vi "_FPGA_ConjSelector.vi"(0 "Conj.InitCyc*2^32":u32, 1 "ConjArr":cluster{"Ratio*2^15":u16, "CycleDiff":u64}[](array[cluster])=[{"Ratio*2^15"=0, "CycleDiff"=0}, {"Ratio*2^15"=0, "CycleDiff"=0}, {"Ratio*2^15"=0, "CycleDiff"=0}, {"Ratio*2^15"=0, "CycleDiff"=0}, {"Ratio*2^15"=0, "CycleDiff"=0}, {"Ratio*2^15"=0, "CycleDiff"=0}, {"Ratio*2^15"=0, "CycleDiff"=0}, {"Ratio*2^15"=0, "CycleDiff"=0}, {"Ratio*2^15"=0, "CycleDiff"=0}, {"Ratio*2^15"=0, "CycleDiff"=0}, {"Ratio*2^15"=0, "CycleDiff"=0}, {"Ratio*2^15"=0, "CycleDiff"=0}, {"Ratio*2^15"=0, "CycleDiff"=0}, {"Ratio*2^15"=0, "CycleDiff"=0}, {"Ratio*2^15"=0, "CycleDiff"=0}, {"Ratio*2^15"=0, "CycleDiff"=0}], 2 "Init_strobe":bool, 5 "ConjSize-1":u8, 9 "1/DeCyc*2^8":u32, 11 "RfCyc_in":u64, 12 "Mode":bool=TRUE) -> (3 "LastConj":bool, 4 "ConjIndex":u8, 6 "Initialising?":bool, 10 "Not Conj?":bool, 14 "Cross Conj?":bool, 15 "RfCyc_out":u64)   [LabVIEW 2018]
uses:
  <instrlib>/_niInstr/Basic Elements/v1/FPGA/Private/Count Down U16.vi
  <instrlib>/_niInstr/Basic Elements/v1/FPGA/niInstr Basic Elements v1 FPGA.lvlib
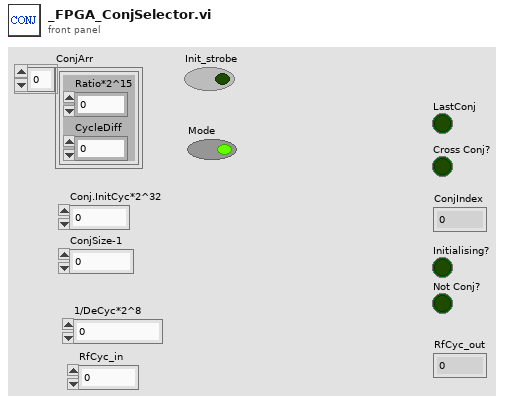
[diagram p1: front panel]
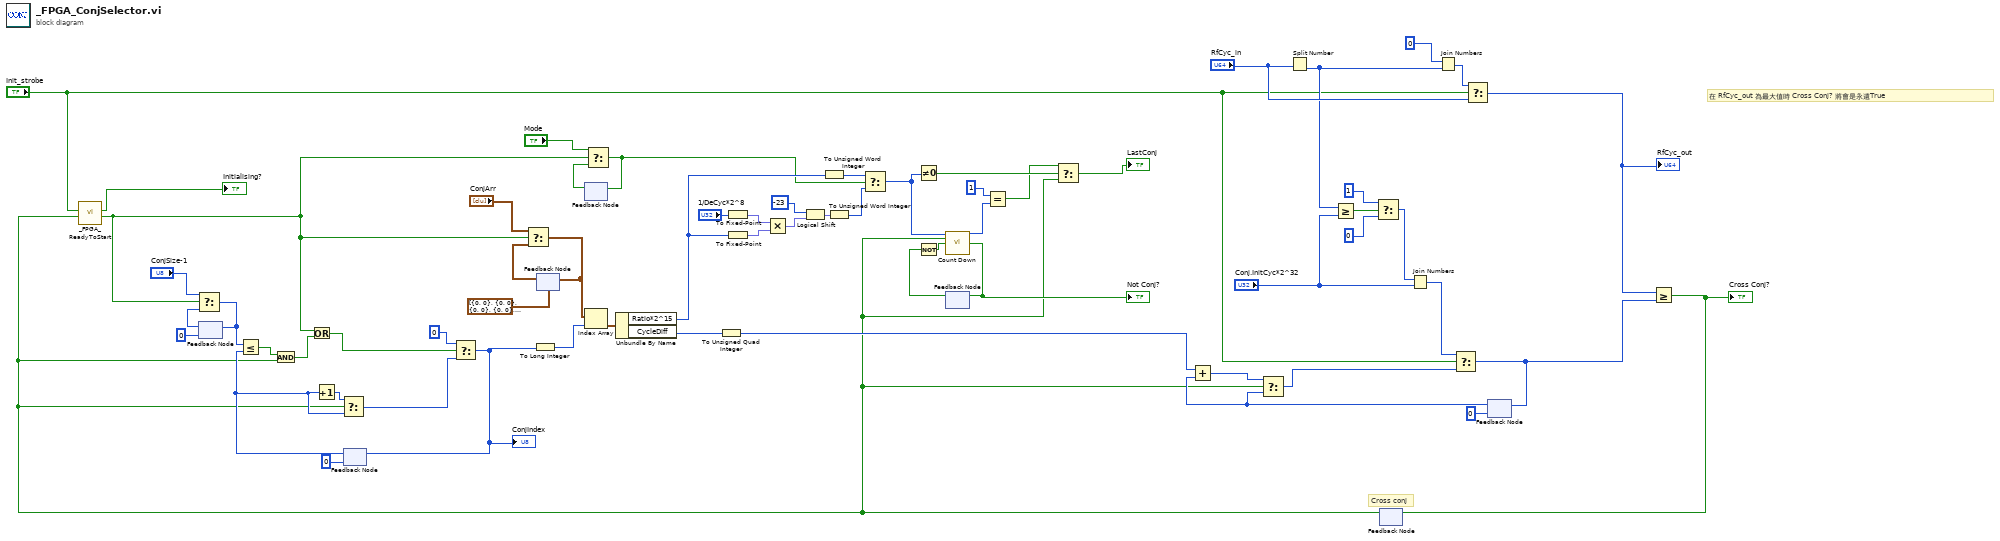
[diagram p0: block diagram]
diagram:
  # "在 RfCyc_out 為最大值時 Cross Conj? 將會是永遠True"
  # "Cross conj"
  n1 = feedback #1(u8 0 ("ConjSize-1")) -> (w35:u8)
  n2 = feedback #2(u8 0) -> (w53:u8)
  n3 = Increment(x=w53) -> (x+1=w54:u8)
  n4 = feedback #3(cluster{"Ratio*2^15":u16, "CycleDiff":u64}[] [{"Ratio*2^15"=0, "CycleDiff"=0}, {"Ratio*2^15"=0, "CycleDiff"=0}, {"Ratio*2^15"=0, "CycleDiff"=0}, {"Ratio*2^15"=0, "CycleDiff"=0}, {"Ratio*2^15"=0, "CycleDiff"=0}, {"Ratio*2^15"=0, "CycleDiff"=0}, {"Ratio*2^15"=0, "CycleDiff"=0}, {"Ratio*2^15"=0, "CycleDiff"=0}, {"Ratio*2^15"=0, "CycleDiff"=0}, {"Ratio*2^15"=0, "CycleDiff"=0}, {"Ratio*2^15"=0, "CycleDiff"=0}, {"Ratio*2^15"=0, "CycleDiff"=0}, {"Ratio*2^15"=0, "CycleDiff"=0}, {"Ratio*2^15"=0, "CycleDiff"=0}, {"Ratio*2^15"=0, "CycleDiff"=0}, {"Ratio*2^15"=0, "CycleDiff"=0}] ("ConjArr")) -> (w49:cluster{"Ratio*2^15":u16, "CycleDiff":u64}[])
  n5 = feedback #4() -> (w5:bool)  [unwired: 1 in]
  n6 = To Fixed-Point(number="1/DeCyc*2^8") -> (fixed-point=w43:fxp<+,32,32>)  [unwired: 1 in]
  n7 = feedback #5() -> (w38:bool)  [unwired: 1 in]
  n8 = Not(x=w38) -> (.not. x?=w39:bool)
  n9 = Split Number(x="RfCyc_in") -> (lo(x)=w31:u32)  [unwired: 1 out]
  n10 = Greater Or Equal?(x=w31, y="Conj.InitCyc*2^32") -> (x >= y?=w29:bool)
  n11 = Select(t=u32 1 ("hi"), s=w29, f=u32 0 ("hi(x)")) -> (s? t:f=w26:u32)
  n12 = feedback #6() -> (w13:bool)  [unwired: 1 in]
  n13 = call "_FPGA_ReadyToStart.vi"("Start_strobe_in"=w13, "Ready_latch_in"="Init_strobe") -> ("Trigger_strobe_out"=w3:bool, "Ready?"=→"Initialising?":bool)  [unwired: 8 in]
  n14 = Select(t="ConjSize-1", s=w3, f=w35) -> (s? t:f=w36:u8)
  n15 = feedback-in #1(w36) -> ()
  n16 = Less Or Equal?(x=w36, y=w53) -> (x <= y?=w56:bool)
  n17 = And(x=w56, y=w13) -> (x .and. y?=w41:bool)
  n18 = Or(x=w3, y=w41) -> (x .or. y?=w33:bool)
  n19 = Select(t=w54, s=w13, f=w53) -> (s? t:f=w51:u8)
  n20 = Select(t=u8 0, s=w33, f=w51) -> (s? t:f=w42:u8)
  "ConjIndex" <- w42
  n21 = feedback-in #2(w42) -> ()
  n22 = Select(t="ConjArr", s=w3, f=w49) -> (s? t:f=w40:cluster{"Ratio*2^15":u16, "CycleDiff":u64}[])
  n23 = To Long Integer(number=w42) -> (32bit integer=w57:i32)
  n24 = feedback-in #3(w40) -> ()
  n25 = Index Array(array=w40, index=w57) -> (element=w58:cluster{"Ratio*2^15":u16, "CycleDiff":u64})
  n26 = Select(t="Mode", s=w3, f=w5) -> (s? t:f=w6:bool)
  n27 = feedback-in #4(w6) -> ()
  n28 = Unbundle By Name(w58) -> ("Ratio*2^15"=w8:u16, "CycleDiff"=w59:u64)
  n29 = To Unsigned Quad Integer(1:w59) -> (0:w34:u64)
  n30 = To Fixed-Point(number=w8) -> (fixed-point=w60:fxp<+,16,16>)  [unwired: 1 in]
  n31 = Multiply(x=w43, y=w60) -> (x*y=w61:fxp<+,48,48>)
  n32 = Logical Shift(y=i16 -23, x=w61) -> (x << y=w63:fxp<+,48,48>)
  n33 = To Unsigned Word Integer(number=w8) -> (unsigned 16bit integer=w11:u16)
  n34 = To Unsigned Word Integer(number=w63) -> (unsigned 16bit integer=w12:u16)
  n35 = Select(t=w11, s=w6, f=w12) -> (s? t:f=w9:u16)
  n36 = Not Equal To 0?(x=w9) -> (x != 0?=w17:bool)
  n37 = call-poly <instrlib>:"Count Down.vi"("count in"=w9, "load"=w13, "decrement"=w39) -> ("count out"=w19:u16, "terminal count"=w14:bool)  [unwired: 11 in]
  "Not Conj?" <- w14
  n38 = feedback-in #5(w14) -> ()
  n39 = Equal?(x=u16 1, y=w19) -> (x = y?=w16:bool)
  n40 = Select(t=w16, s=w17, f=w13) -> (s? t:f=→"LastConj":bool)
  n41 = Join Numbers(hi=w26, lo="Conj.InitCyc*2^32") -> ((hi.lo)=w25:u64)
  n42 = Join Numbers(hi=u32 0 ("hi(x)"), lo=w31) -> ((hi.lo)=w46:u64)
  n43 = Select(t=w46, s="Init_strobe", f="RfCyc_in") -> (s? t:f=w24:u64)
  "RfCyc_out" <- w24
  n44 = feedback #7(u64 0) -> (w50:u64)
  n45 = Add(x=w34, y=w50) -> (x+y=w55:u64)
  n46 = Select(t=w55, s=w13, f=w50) -> (s? t:f=w48:u64)
  n47 = Select(t=w25, s="Init_strobe", f=w48) -> (s? t:f=w45:u64)
  n48 = feedback-in #7(w45) -> ()
  n49 = Greater Or Equal?(x=w24, y=w45) -> (x >= y?=w44:bool)
  "Cross Conj?" <- w44
  n50 = feedback-in #6(w44) -> ()
